vi "CheckState.vi"(8 "Error In":errorcluster, 10 "With sound?":bool, 11 "Droid in":refnum<class "Droid.lvclass">) -> (0 "Error Out":errorcluster, 3 "Droid out":refnum<class "Droid.lvclass">)   [LabVIEW 2021, in "Droid.lvclass"]
uses:
  Droid.lvclass
  Droid.lvclass/Droid.ctl
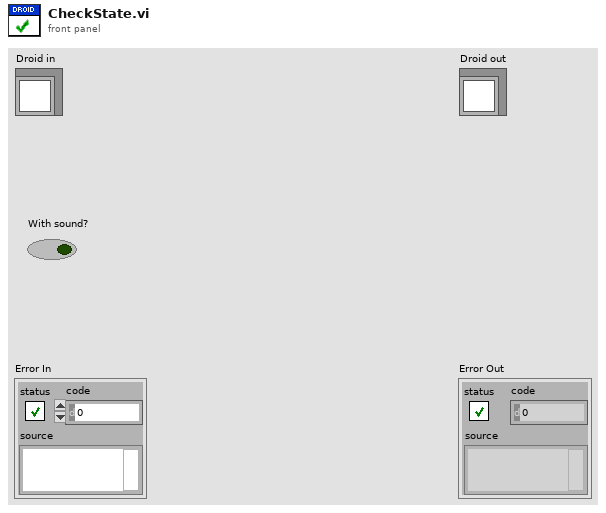
[diagram p1: front panel]
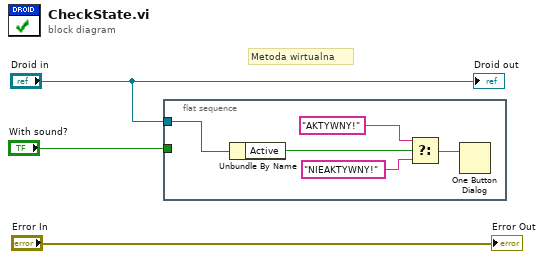
[diagram p0: block diagram]
diagram:
  # "Metoda wirtualna"
  n1 = flat-sequence {
    tunnel: "With sound?" -> [_]
    tunnel: "Droid in" -> [w8]
    frame #0 {
      n2 = Unbundle By Name(w8) -> ("Active"=w7:bool)
      n3 = Select(t="AKTYWNY!", s=w7, f="NIEAKTYWNY!") -> (s? t:f=w4:string)
      n4 = One Button Dialog(message=w4) -> ()  [unwired: 1 in, 1 out]
    }
  }
  "Error Out" <- "Error In"
  "Droid out" <- "Droid in"
